vi "FGV.vi"(6 "Action":T1, 11 "Param in":T3) -> (3 "Param out":T2)   [LabVIEW 2023]
uses:
  Param in.ctl
  Param out.ctl
  enum_FGV.ctl
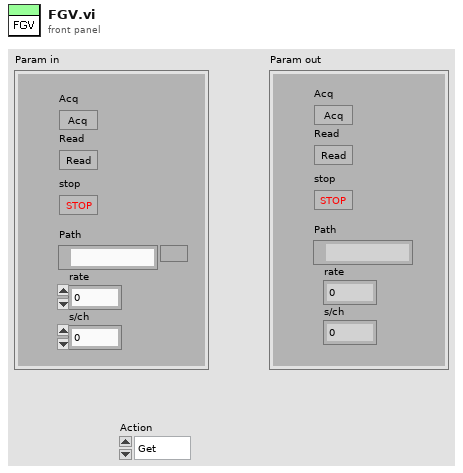
[diagram p1: front panel]
types:
  T1 = typedef "enum_FGV.ctl" = enum16{"Get", "Set"}
  T2 = typedef "Param out.ctl" = cluster{"Acq":bool, "stop":bool, "Path":path, "rate":dbl, "s/ch":dbl, "Read":bool}
  T3 = typedef "Param in.ctl" = cluster{"Acq":bool, "stop":bool, "Path":path, "rate":dbl, "s/ch":dbl, "Read":bool}
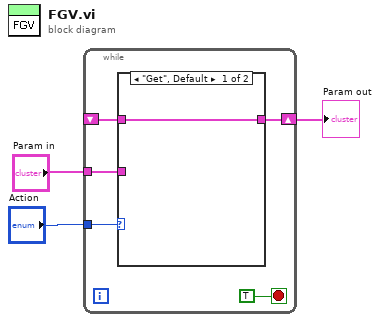
[diagram p0: block diagram]
diagram:
  n1 = while {
    tunnel: "Action" -> [w7]
    tunnel: "Param in" -> [w5]
    shift-right: [w6] -> w2
    shift-left: _ -> [w4]
    stop <- TRUE stop-if-true
    n2 = case shown="\"Get\", Default" w7 {
      tunnel: [w9 w10] -> w6
      tunnel: w5 -> [_ w10]
      tunnel: w4 -> [w9 _]
      frame "Get", Default {
      }
      frame "Set" {
      }
    }
  }
  "Param out" <- w2
